vi "Test All.vi"(11 "Error in":errorcluster) -> (15 "Error out":errorcluster)   [LabVIEW 2020, in "CelsiusToFarenheitTests.lvlib"]
doc: "This vi runs all the test cases for the Celsius to Fahrenheit assignment. Also the test report gets saved as a xml format.\n\n* USES *\nDrona, G-CLI and Caraya"
uses:
  CelsiusToFarenheitTests.lvlib
  <vilib>/addons/_JKI Toolkits/Caraya/classes/Test Suite/Define Test Suite (JUnit Report).vi
  <vilib>/Utility/error.llb/Error Cluster From Error Code.vi
  <vilib>/ErrorRing/Error Ring.xnode
  <vilib>/addons/_JKI Toolkits/Caraya/classes/Test Suite/Test Suite.lvclass
  <vilib>/addons/_JKI Toolkits/Caraya/classes/Test/Test.lvclass
  <vilib>/Wiresmith Technology/G CLI/CLI Class/CLI.lvclass
  <vilib>/addons/_JKI Toolkits/Caraya/classes/Test Result/Test Result.lvclass
panel:
  # "TESTING ALL TEST CASES FOR CELSIUS TO FAHRENHEIT"
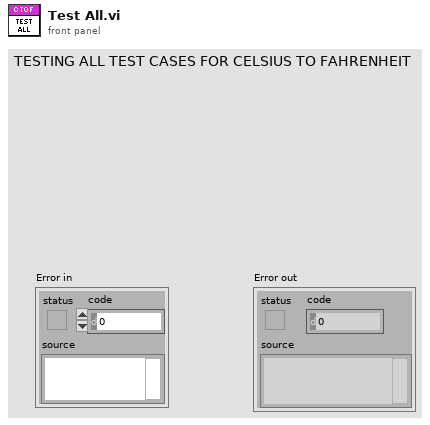
[diagram p1: front panel]
types:
  T1 = typedef "Caraya.lvlib/Test Result.lvclass/Node Results.ctl" = cluster{"Node":T2, "Assertions":T4[]}
  T2 = typedef "Caraya.lvlib/Test Result.lvclass/Test Node.ctl" = cluster{"Test Registration":T3, "Defined":bool, "Passed":bool}
  T3 = typedef "Caraya.lvlib/Test Result.lvclass/Test Registration Data.ctl" = cluster{"Name":string, "Call Chain":string[], "Time Stamp":timestamp, "Test ID":string, "Caller ID":string}
  T4 = typedef "Caraya.lvlib/Test Result.lvclass/Assert Event Data.ctl" = cluster{"Name":string, "Passed":bool, "Call Chain":string[], "Test Error":errorcluster, "Time Stamp":timestamp, "Unique Assert ID":string, "Test ID":string, "Execution time (s)":dbl, "Verbose Explanation":string}
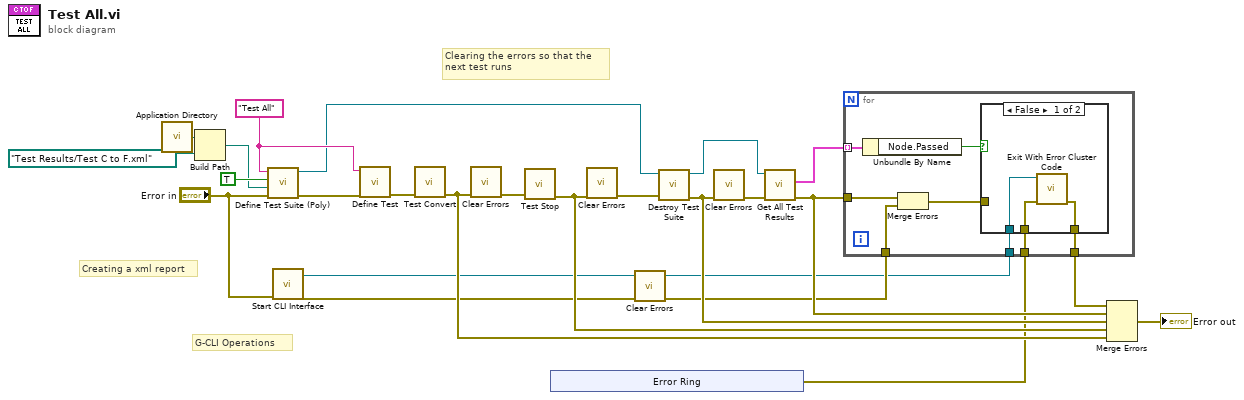
[diagram p0: block diagram]
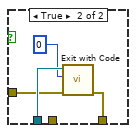
[diagram p2: hidden frame]
diagram:
  w19 = "Test All" ("Label (VI Title)")
  # "G-CLI Operations"
  # "Creating a xml report"
  # "Clearing the errors so that the\nnext test runs"
  n1 = call <vilib>:"Application Directory.vi"() -> ("Application Directory"=w24:path)
  n2 = Build Path(base path=w24, name or relative path=path "Test Results/Test C to F.xml") -> (appended path=w21:path)
  n3 = call-poly <vilib>:"Define Test Suite (Poly).vi"("error in (no error)"="Error in", "Report Path"=w21, "Interactive"=TRUE, "Label (VI Title)"=w19) -> ("error out"=w20:errorcluster, "Test Suite"=w18:refnum<class "Test Suite.lvclass">)  [unwired: 6 in]
  n4 = call <vilib>:"Start CLI Interface.vi"("error in (no error)"="Error in") -> ("error out"=w2:errorcluster, "CLI out"=w1:refnum<class "CLI.lvclass">)  [unwired: 7 in, 2 out]
  n5 = call <vilib>:"Define Test.vi"("error in (no error)"=w20, "Label (VI Title)"=w19) -> ("error out"=w17:errorcluster)  [unwired: 9 in]
  n6 = call "Test Convert.vi"("Error in"=w17) -> ("Error out"=w14:errorcluster)  [unwired: 14 in]
  n7 = call <vilib>:"Clear Errors.vi"("error in (no error)"=w14) -> ("error out"=w16:errorcluster)  [unwired: 5 in, 1 out]
  n8 = call "Test Stop.vi"("Error in"=w16) -> ("Error out"=w13:errorcluster)  [unwired: 14 in]
  n9 = xnode "Error Ring"() -> ("error out"=w3:errorcluster)
  n10 = call <vilib>:"Clear Errors.vi"("error in (no error)"=w13) -> ("error out"=w15:errorcluster)  [unwired: 5 in, 1 out]
  n11 = call <vilib>:"Clear Errors.vi"("error in (no error)"=w2) -> ("error out"=w4:errorcluster)  [unwired: 5 in, 1 out]
  n12 = call-dynamic "Destroy Test Suite.vi"("error in (no error)"=w15, "Test Suite in"=w18) -> ("error out"=w7:errorcluster, "Test Suite Results"=w9:refnum<class "Test Result.lvclass">)  [unwired: 8 in]
  n13 = call <vilib>:"Clear Errors.vi"("error in (no error)"=w7) -> ("error out"=w8:errorcluster)  [unwired: 5 in, 1 out]
  n14 = call <vilib>:"Get All Test Results.vi"("error in (no error)"=w8, "Test Result in"=w9) -> ("error out"=w5:errorcluster, "Test Results"=w10:T1[])  [unwired: 7 in, 1 out]
  n15 = for {
    tunnel: w10 -> [w32] mode=indexing
    tunnel: w1 -> [w30]
    tunnel: [w29] -> w6
    tunnel: w5 -> [w28]
    tunnel: w4 -> [w27]
    tunnel: w3 -> [w25]
    n16 = Unbundle By Name(w32) -> ("Node.Passed"=w31:bool)
    n17 = Merge Errors(w28, w27) -> (w26:errorcluster)
    n18 = case shown="False" w31 {
      tunnel: w30 -> [w35 w39]
      tunnel: [w34 w37] -> w29
      tunnel: w26 -> [_ w36]
      tunnel: w25 -> [w33 _]
      frame False {
        n19 = call <vilib>:"Exit With Error Cluster Code.vi"("error in (no error)"=w33, "CLI in"=w35) -> ("error out"=w34:errorcluster)  [unwired: 9 in]
      }
      frame True {
        n20 = call <vilib>:"Exit with Code.vi"("error in (no error)"=w36, "Exit Code (0)"=0, "CLI in"=w39) -> ("error out"=w37:errorcluster)  [unwired: 8 in]
      }
    }
  }
  n21 = Merge Errors(w6, w5, w7, w13, w14) -> (→"Error out":errorcluster)
